vi "Activate-Deactivate Analog Channels.vi"(8 "error in (no error)":errorcluster, 10 "Active Channel(s)":T1[](array[typedef]), 11 "VISA resource name":refnum<visa-resource-name>) -> (0 "error out":errorcluster, 3 "VISA resource name out":refnum<visa-resource-name>)   [LabVIEW 2018, in "DPO4104.lvlib" / "DPO4104.lvclass"]
doc: "This VI sends commands to activate channels specified in the Active Channel(s) input."
uses:
  DPO4104.lvclass
  PPLs/Oscilloscope/Parent/Oscilloscope.lvlibp/Custom Controls/Analog Channels.ctl
  <instrlib>/Tektronix DPO MSO 2000 4000 Series/Tektronix DPO MSO 2000 4000 Series.lvlib
  PPLs/Oscilloscope/Parent/Oscilloscope.lvlibp
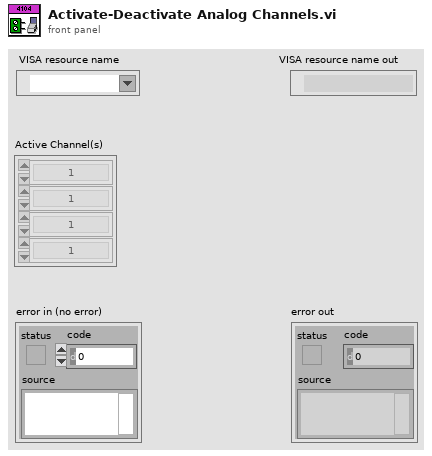
[diagram p1: front panel]
types:
  T1 = typedef "Oscilloscope.lvlibp/Analog Channels.ctl" = enum16{"1", "2", "3", "4", "5", "6", "7", "8", "9", "10", "11", "12", "13", "14", "15", "16"}
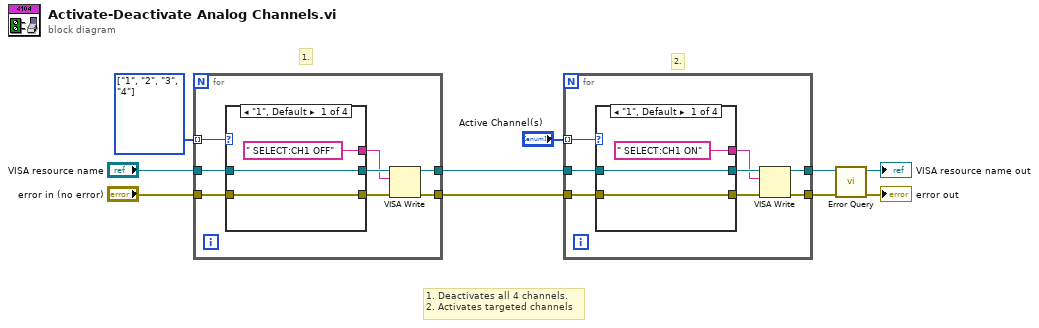
[diagram p0: block diagram]
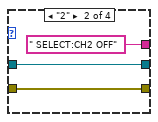
[diagram p2: hidden frame]
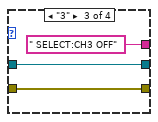
[diagram p3: hidden frame]
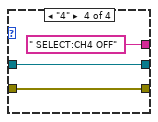
[diagram p4: hidden frame]
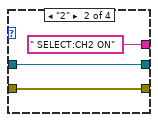
[diagram p5: hidden frame]
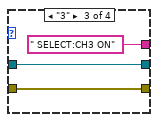
[diagram p6: hidden frame]
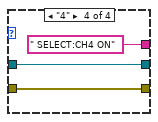
[diagram p7: hidden frame]
diagram:
  w3 = T1[] [enum."1", enum."2", enum."3", enum."4"] items=["1", "2", "3", "4", "5", "6", "7", "8", "9", "10", "11", "12", "13", "14", "15", "16"] ("Active Channel(s)")
  # "1. Deactivates all 4 channels.\n2. Activates targeted channels"
  # "2."
  # "1."
  n1 = for {
    tunnel: w3 -> [w18] mode=indexing
    tunnel: "error in (no error)" -> [w17]
    tunnel: "VISA resource name" -> [w16]
    tunnel: [w12] -> w5
    tunnel: [w11] -> w4
    n2 = case shown="\"1\", Default" w18 {
      tunnel: w17 -> [w20 w23 w26 w29]
      tunnel: w16 -> [w19 w22 w25 w28]
      tunnel: [" SELECT:CH1 OFF" " SELECT:CH2 OFF" " SELECT:CH3 OFF" " SELECT:CH4 OFF"] -> w13
      tunnel: [w20 w23 w26 w29] -> w15
      tunnel: [w19 w22 w25 w28] -> w14
      frame "1", Default {
      }
      frame "2" {
      }
      frame "3" {
      }
      frame "4" {
      }
    }
    n3 = VISA Write(VISA resource name=w14, write buffer=w13, error in (no error)=w15) -> (VISA resource name out=w11:refnum<visa-resource-name>, error out=w12:errorcluster)  [unwired: 1 out]
  }
  n4 = for {
    tunnel: "Active Channel(s)" -> [w38] mode=indexing
    tunnel: w5 -> [w37]
    tunnel: w4 -> [w36]
    tunnel: [w32] -> w8
    tunnel: [w31] -> w7
    n5 = case shown="\"1\", Default" w38 {
      tunnel: w37 -> [w40 w43 w46 w49]
      tunnel: w36 -> [w39 w42 w45 w48]
      tunnel: [" SELECT:CH1 ON" " SELECT:CH2 ON" " SELECT:CH3 ON" " SELECT:CH4 ON"] -> w33
      tunnel: [w40 w43 w46 w49] -> w35
      tunnel: [w39 w42 w45 w48] -> w34
      frame "1", Default {
      }
      frame "2" {
      }
      frame "3" {
      }
      frame "4" {
      }
    }
    n6 = VISA Write(VISA resource name=w34, write buffer=w33, error in (no error)=w35) -> (VISA resource name out=w31:refnum<visa-resource-name>, error out=w32:errorcluster)  [unwired: 1 out]
  }
  n7 = call <instrlib>:"Error Query.vi"("error in (no error)"=w8, "VISA resource name"=w7) -> ("error out"=→"error out":errorcluster, "VISA resource name out"=→"VISA resource name out":refnum<visa-resource-name>)  [unwired: 6 in, 2 out]
